vi "Bind Insert Command Parameters.vi"(8 "Error In (no error)":errorcluster, 10 "Record":variant, 11 "SQL Statement In":refnum<class "SQL Statement.lvclass">) -> (0 "Error Out":errorcluster, 3 "SQL Statement Out":refnum<class "SQL Statement.lvclass">)   [LabVIEW 2023, in "SQLite DB Operator.lvclass"]
uses:
  SQLite DB Operator.lvclass
  <vilib>/drjdpowell/SQLite Library/SQL Statement/SQL Statement.lvclass
  DB Records/Expenses Tracker Record/Public/Ctrls/Category.ctl
  <vilib>/drjdpowell/SQLite Library/SQL Statement/SQL Statement.lvclass/SQL Statement.ctl
  DB Records/Expenses Tracker Record/Public/Ctrls/Subcategory.ctl
  DB Records/Expenses Tracker Record/Public/Ctrls/Balance.ctl
  DB Records/Expenses Tracker Record/Public/Ctrls/Cycle.ctl
  DB Records/Expenses Tracker Record/Public/Ctrls/Transaction.ctl
  <vilib>/drjdpowell/SQLite Library/SQL Statement/Bind Text.vi
  <vilib>/drjdpowell/SQLite Library/SQL Statement/Bind Integer.vi
  <vilib>/drjdpowell/SQLite Library/SQL Statement/Bind Null.vi
  <vilib>/drjdpowell/SQLite Library/SQL Statement/Bind Timestamp (Real).vi
  <vilib>/drjdpowell/SQLite Library/SQL Statement/Bind Real.vi
  <vilib>/drjdpowell/SQLite Library/SQL Statement/Error Message.vi
  DB Records/Expenses Tracker Record/Expenses Tracker Record.lvclass
  <vilib>/Utility/Data Type/NI_Data Type.lvlib
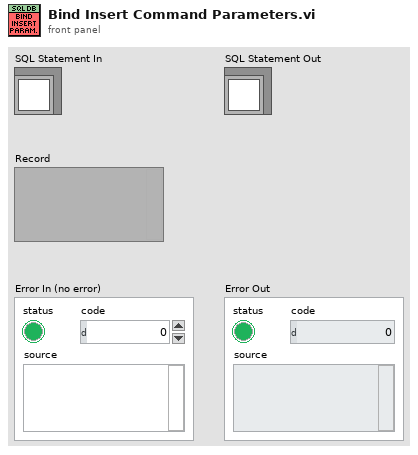
[diagram p1: front panel]
types:
  T1 = typedef "Expenses Tracker Record.lvclass/Category.ctl" = cluster{"ID":u32, "Name":string}
  T2 = typedef "Expenses Tracker Record.lvclass/Subcategory.ctl" = cluster{"ID":u32, "Name":string, "Category":u32}
  T3 = typedef "Expenses Tracker Record.lvclass/Balance.ctl" = cluster{"ID":u8, "Value":dbl, "Last_update":timestamp}
  T4 = typedef "Expenses Tracker Record.lvclass/Cycle.ctl" = cluster{"ID":u32, "Name":string, "Day_of_occurence":u8, "Description":string}
  T5 = typedef "Expenses Tracker Record.lvclass/Transaction.ctl" = cluster{"ID":u32, "Name":string, "Is_income":bool, "Value":dbl, "Amount":dbl, "Total":dbl, "Date_of_entry":timestamp, "Date":timestamp, "Last_update":timestamp, "Category":u32, "Subcategory":u32, "Cycle":u32, "Description":string}
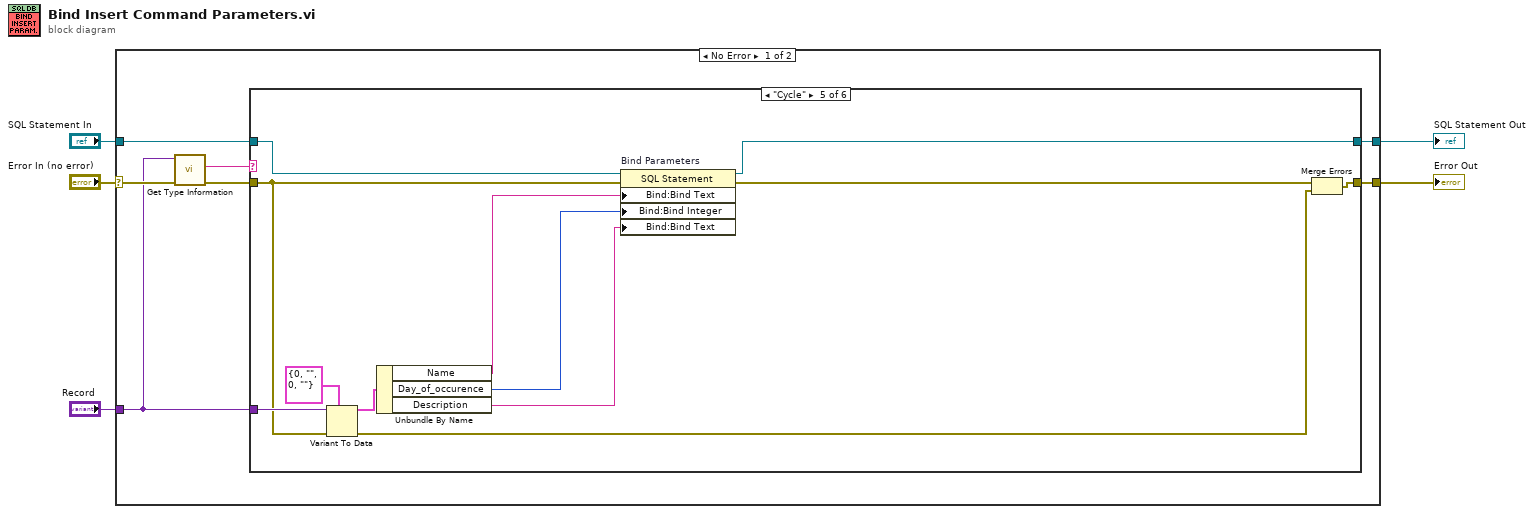
[diagram p0: block diagram]
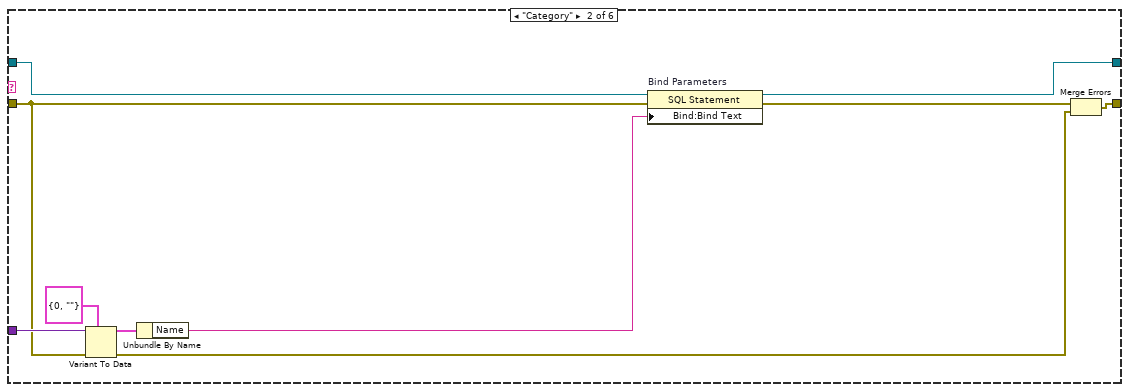
[diagram p3: hidden frame]
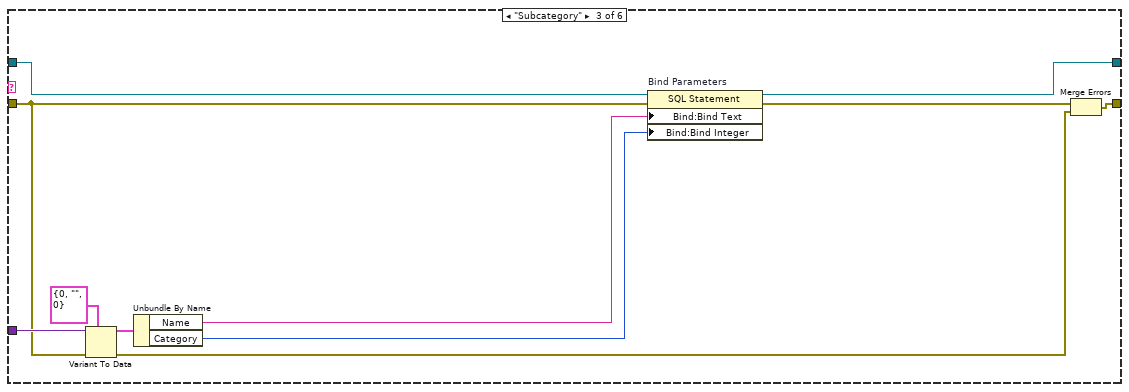
[diagram p4: hidden frame]
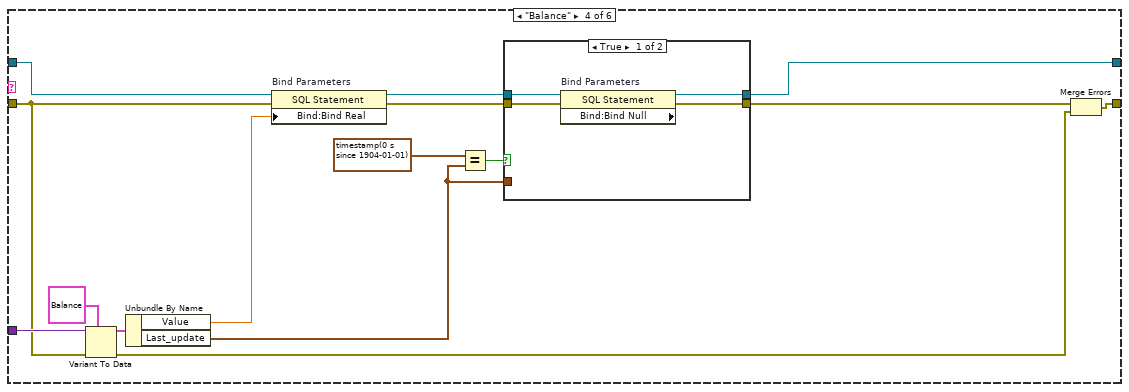
[diagram p5: hidden frame]
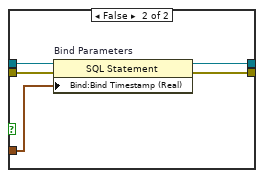
[diagram p6: hidden frame]
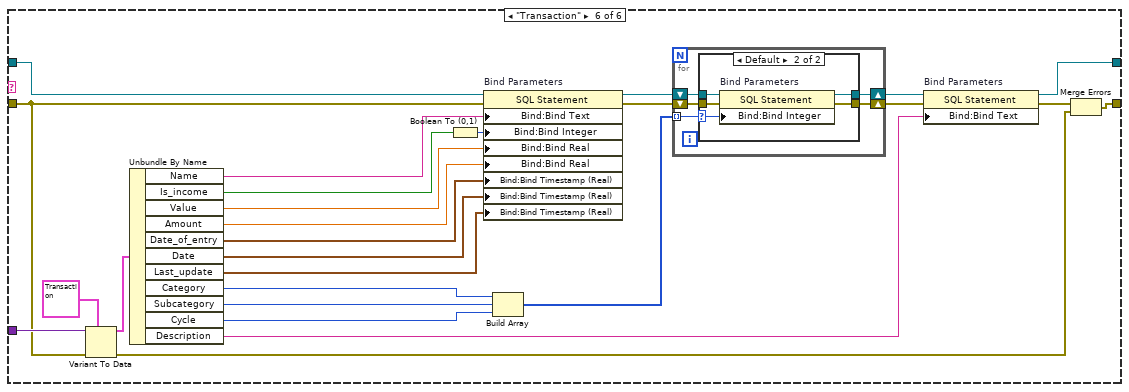
[diagram p7: hidden frame]
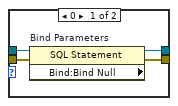
[diagram p8: hidden frame]
diagram:
  n1 = case shown="No Error" "Error In (no error)" {
    selector: "Error In (no error)" -> [w9 w112]
    tunnel: "SQL Statement In" -> [w12 w113]
    tunnel: [w11 w112] -> w4
    tunnel: [w10 w113] -> w3
    tunnel: "Record" -> [w8 _]
    frame No Error {
      n2 = call <vilib>:"Get Type Information.vi"("error in (no error)"=w9, "variant"=w8) -> ("error out"=w6:errorcluster, "name"=w7:string)  [unwired: 5 in, 3 out]
      n3 = case shown="\"Cycle\"" w7 {
        tunnel: w8 -> [_ w24 w35 w50 w71 w97]
        tunnel: [w13 w23 w34 w40 w62 w79] -> w10
        tunnel: [w14 w18 w29 w46 w67 w93] -> w11
        tunnel: w12 -> [w13 w15 w26 w43 w64 w72]
        tunnel: w6 -> [w14 w16 w27 w44 w65 w73]
        frame Default {
        }
        frame "Category" {
          n4 = Variant To Data(error in=w16, type=T1 {"ID"=0, "Name"=""} ("Category"), Variant=w24) -> (data=w21:T1, error out=w17:errorcluster)
          n5 = Unbundle By Name(w21) -> ("Name"=w19:string)
          n6 = property on="Bind Parameters" class="SQL Statement"(reference=w15, error in=w16, "Bind:Bind Text"=w19) -> (reference out=w23:refnum<class "SQL Statement.lvclass">, error out=w22:errorcluster)
          n7 = Merge Errors(w22, w17) -> (w18:errorcluster)
        }
        frame "Subcategory" {
          n8 = Variant To Data(error in=w27, type=T2 {"ID"=0, "Name"="", "Category"=0} ("Subcategory"), Variant=w35) -> (data=w32:T2, error out=w28:errorcluster)
          n9 = Unbundle By Name(w32) -> ("Name"=w30:string, "Category"=w25:u32)
          n10 = property on="Bind Parameters" class="SQL Statement"(reference=w26, error in=w27, "Bind:Bind Text"=w30, "Bind:Bind Integer"=w25) -> (reference out=w34:refnum<class "SQL Statement.lvclass">, error out=w33:errorcluster)
          n11 = Merge Errors(w33, w28) -> (w29:errorcluster)
        }
        frame "Balance" {
          n12 = Variant To Data(error in=w44, type=T3 {"ID"=0, "Value"=0.0, "Last_update"=timestamp(0 s since 1904-01-01)} ("Balance"), Variant=w50) -> (data=w49:T3, error out=w45:errorcluster)
          n13 = Unbundle By Name(w49) -> ("Value"=w47:dbl, "Last_update"=w36:timestamp)
          n14 = property on="Bind Parameters" class="SQL Statement"(reference=w43, error in=w44, "Bind:Bind Real"=w47) -> (reference out=w41:refnum<class "SQL Statement.lvclass">, error out=w42:errorcluster)
          n15 = Equal?(x=timestamp(0 s since 1904-01-01), y=w36) -> (x = y?=w38:bool)
          n16 = case shown="True" w38 {
            tunnel: w42 -> [w54 w59]
            tunnel: w41 -> [w53 w58]
            tunnel: [w52 w57] -> w40
            tunnel: [w51 w56] -> w39
            tunnel: w36 -> [_ w55]
            frame True {
              n17 = property on="Bind Parameters" class="SQL Statement" props=["Bind:Bind Null"](reference=w53, error in=w54) -> (reference out=w52:refnum<class "SQL Statement.lvclass">, error out=w51:errorcluster)  [unwired: 1 out]
            }
            frame False {
              n18 = property on="Bind Parameters" class="SQL Statement"(reference=w58, error in=w59, "Bind:Bind Timestamp (Real)"=w55) -> (reference out=w57:refnum<class "SQL Statement.lvclass">, error out=w56:errorcluster)
            }
          }
          n19 = Merge Errors(w39, w45) -> (w46:errorcluster)
        }
        frame "Cycle" {
          n20 = Variant To Data(error in=w65, type=T4 {"ID"=0, "Name"="", "Day_of_occurence"=0, "Description"=""} ("Cycle"), Variant=w71) -> (data=w70:T4, error out=w66:errorcluster)
          n21 = Unbundle By Name(w70) -> ("Name"=w68:string, "Day_of_occurence"=w61:u8, "Description"=w60:string)
          n22 = property on="Bind Parameters" class="SQL Statement"(reference=w64, error in=w65, "Bind:Bind Text"=w68, "Bind:Bind Integer"=w61, "Bind:Bind Text"=w60) -> (reference out=w62:refnum<class "SQL Statement.lvclass">, error out=w63:errorcluster)
          n23 = Merge Errors(w63, w66) -> (w67:errorcluster)
        }
        frame "Transaction" {
          n24 = Variant To Data(error in=w73, type=T5 {"ID"=0, "Name"="", "Is_income"=FALSE, "Value"=0.0, "Amount"=0.0, "Total"=0.0, "Date_of_entry"=timestamp(0 s since 1904-01-01), "Date"=timestamp(0 s since 1904-01-01), "Last_update"=timestamp(0 s since 1904-01-01), "Category"=0, "Subcategory"=0, "Cycle"=0, "Description"=""} ("Transaction"), Variant=w97) -> (data=w96:T5, error out=w92:errorcluster)
          n25 = Unbundle By Name(w96) -> ("Name"=w94:string, "Is_income"=w86:bool, "Value"=w90:dbl, "Amount"=w91:dbl, "Date_of_entry"=w89:timestamp, "Date"=w88:timestamp, "Last_update"=w87:timestamp, "Category"=w77:u32, "Subcategory"=w76:u32, "Cycle"=w75:u32, "Description"=w78:string)
          n26 = Boolean To (0,1)(Boolean=w86) -> (0, 1=w85:i16)
          n27 = property on="Bind Parameters" class="SQL Statement"(reference=w72, error in=w73, "Bind:Bind Text"=w94, "Bind:Bind Integer"=w85, "Bind:Bind Real"=w90, "Bind:Bind Real"=w91, "Bind:Bind Timestamp (Real)"=w89, "Bind:Bind Timestamp (Real)"=w88, "Bind:Bind Timestamp (Real)"=w87) -> (reference out=w83:refnum<class "SQL Statement.lvclass">, error out=w84:errorcluster)
          n28 = Build Array(w77, w76, w75) -> (w74:u32[])
          n29 = for {
            shift-right: [w99] -> w81
            shift-left: w84 -> [w102]
            shift-right: [w100] -> w82
            shift-left: w83 -> [w101]
            tunnel: w74 -> [w98] mode=indexing
            n30 = case shown="Default" w98 {
              selector: w98 -> [_ w107]
              tunnel: w102 -> [w106 w111]
              tunnel: w101 -> [w105 w110]
              tunnel: [w104 w109] -> w100
              tunnel: [w103 w108] -> w99
              frame 0 {
                n31 = property on="Bind Parameters" class="SQL Statement" props=["Bind:Bind Null"](reference=w105, error in=w106) -> (reference out=w104:refnum<class "SQL Statement.lvclass">, error out=w103:errorcluster)  [unwired: 1 out]
              }
              frame Default {
                n32 = property on="Bind Parameters" class="SQL Statement"(reference=w110, error in=w111, "Bind:Bind Integer"=w107) -> (reference out=w109:refnum<class "SQL Statement.lvclass">, error out=w108:errorcluster)
              }
            }
          }
          n33 = property on="Bind Parameters" class="SQL Statement"(reference=w82, error in=w81, "Bind:Bind Text"=w78) -> (reference out=w79:refnum<class "SQL Statement.lvclass">, error out=w80:errorcluster)
          n34 = Merge Errors(w80, w92) -> (w93:errorcluster)
        }
      }
    }
    frame Error {
    }
  }
  "Error Out" <- w4
  "SQL Statement Out" <- w3
